vi "Begin.vi"(8 "error in":errorcluster) -> (0 "error out":errorcluster)   [LabVIEW 2015]
doc: "Called before other user functions, this VI is expected to open initial I/O refnums, load in file data, and do all program initialization. Notice that the <B>error out</B> terminal is simply used for data flow. Wiring it to other structures or subVIs ensures that this VI runs first."
uses:
  <vilib>/Rock Robotics/WPI/DriverStation/WPI_DriverStationRobotMode2.ctl
  <vilib>/Rock Robotics/WPI/Joystick/WPI_JoystickDeviceEnum.ctl
  <vilib>/Rock Robotics/SystemInterfaces/DIO/FPGA_DIOChannel.ctl
  <vilib>/Rock Robotics/SystemInterfaces/DIO/FPGA_DIORelayChannel.ctl
  <vilib>/Rock Robotics/WPI/Solenoid/WPI_SolenoidChannel.ctl
  <vilib>/Rock Robotics/SystemInterfaces/DIO/FPGA_DIOPWMChannel.ctl
  <vilib>/Rock Robotics/SystemInterfaces/spilib/spi_bus.ctl
  Robot Global Data.vi
  <vilib>/Rock Robotics/Network Tables/NT Write String Array.vi
  <vilib>/Rock Robotics/WPI/Switch/WPI_SwitchOpenLimit.vi
  <vilib>/Rock Robotics/WPI/Solenoid/WPI_SolenoidOpenDouble.vi
  <vilib>/Rock Robotics/WPI/Counter/WPI_CounterDigitalInputToDigitalSource.vi
  <vilib>/Rock Robotics/WPI/MotorControl/WPI_MotorControlOpenCANTalonSRX.vi
  <vilib>/Rock Robotics/WPI/MotorControl/WPI_MotorControlOpen VictorSP.vi
  <vilib>/Rock Robotics/WPI/Gyro/WPI_GyroXRS450_SPI_Open.vi
  <vilib>/Rock Robotics/WPI/Utilities/WPI_GetSetVariantRefNum.vi
  <vilib>/Rock Robotics/WPI/Accelerometer/InternalAccelerometer/WPI_AccelerometerInternalOpen.vi
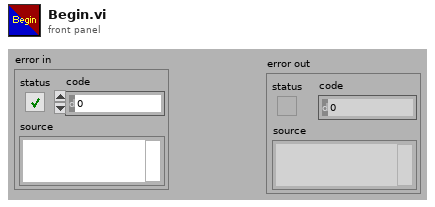
[diagram p1: front panel]
types:
  T1 = typedef "spi_bus.ctl" = enum16{"SPI On-Board, CS0", "SPI On-Board, CS1", "SPI On-Board, CS2", "SPI On-Board, CS3", "SPI MXP", "Invalid"}
  T2 = typedef "WPI_SolenoidChannel.ctl" = enum8{"Solenoid 0", "Solenoid 1", "Solenoid 2", "Solenoid 3", "Solenoid 4", "Solenoid 5", "Solenoid 6", "Solenoid 7", "Invalid"}
  T3 = typedef "FPGA_DIOPWMChannel.ctl" = enum8{"PWM 0", "PWM 1", "PWM 2", "PWM 3", "PWM 4", "PWM 5", "PWM 6", "PWM 7", "PWM 8", "PWM 9", "PWM MXP 0", "PWM MXP 1", "PWM MXP 2", "PWM MXP 3", "PWM MXP 4", "PWM MXP 5", "PWM MXP 6", "PWM MXP 7", "PWM MXP 8", "PWM MXP 9", "Invalid"}
  T4 = typedef "FPGA_DIOChannel.ctl" = enum8{"DIO 0", "DIO 1", "DIO 2", "DIO 3", "DIO 4", "DIO 5", "DIO 6", "DIO 7", "DIO 8", "DIO 9", "DIO MXP 0", "DIO MXP 1", "DIO MXP 2", "DIO MXP 3", "DIO MXP 4", "DIO MXP 5", "DIO MXP 6", "DIO MXP 7", "DIO MXP 8", "DIO MXP 9", "DIO MXP 10", "DIO MXP 11", "DIO MXP 12", "DIO MXP 13", "DIO MXP 14", "DIO MXP 15", "Invalid"}
  T5 = typedef "FPGA_DIORelayChannel.ctl" = enum8{"Relay 0", "Relay 1", "Relay 2", "Relay 3", "Invalid"}
  T6 = typedef "WPI_JoystickDeviceEnum.ctl" = enum16{"USB 0", "USB 1", "USB 2", "USB 3", "USB 4", "USB 5"}
  T7 = typedef "WPI_DriverStationRobotMode2.ctl" = enum16{"Autonomous Disabled", "Autonomous Enabled", "Teleop Disabled", "Teleop Enabled", "Disconnected", "Finish", "Test Disabled", "Test Enabled", "Emergency Stopped"}
  T8 = typedef "WPI_AccelerometerDevRef.ctl" = cluster{"DevStatus":errorcluster, "Scaling":T9, "Analog Channels":T10, "I2C Bus":T12, "SPI Bus":T1, "Accel Range":T13, "ADXL Axes":T14, "Handle":i32, "Device Address":u8, "Accel Type":enum16{"Analog", "ADXL345 I2C", "ADXL345 SPI", "Internal", "ADXL362 SPI"}}
  T9 = typedef "WPI_AccelerometerScaling.ctl" = cluster{"Gain (VoltsPerG)":dbl, "Center Voltage":dbl}
  T10 = typedef "WPI_AccelerometerAnalogChannels.ctl" = cluster{"X-Axis":T11, "Y-Axis":T11, "Z-Axis":T11}
  T11 = typedef "FPGA_AIChannel.ctl" = enum8{"AI 0", "AI 1", "AI 2", "AI 3", "AI MXP 0", "AI MXP 1", "AI MXP 2", "AI MXP 3", "Invalid"}
  T12 = typedef "i2c_bus.ctl" = enum16{"I2C On-Board", "I2C MXP", "Invalid"}
  T13 = typedef "ADXL345 Range.ctl" = u8
  T14 = typedef "WPI_AccelerometerADXL345 Axes.ctl" = cluster{"X-Axis":bool, "Y-Axis":bool, "Z-Axis":bool}
  T15 = typedef "WPI_CompressorDevRef.ctl" = cluster{"DevStatus":errorcluster, "Pneumatics Control Module":u8}
  T16 = typedef "WPI_MotorControlDeviceRef.ctl" = cluster{"DeviceStatus":errorcluster, "Type":T17, "PWM":cluster{"PWM Channel":T3, "DeadBand":T18}, "CAN":cluster{"Device Number":u8, "Control Mode":T19, "Semaphore":T20, "Max Vout":dbl, "TalonSRX Control Mode":T21}, "Invert":bool}
  T17 = typedef "WPI_MotorControlType.ctl" = enum16{"PWM", "CAN", "CANTalonSRX"}
  T18 = typedef "WPI_PWMDeadband.ctl" = cluster{"Name":string, "maxPositivePwm":i32, "minPositivePwm":i32, "centerPwm":i32, "maxNegativePwm":i32, "minNegativePwm":i32, "angularRange":u16}
  T19 = typedef "WPI_CANJaguar_ControlMode.ctl" = enum8{"Percent VBus", "Current", "Speed", "Position", "Voltage"}
  T20 = typedef "Semaphore RefNum" = refnum<k1>
  T21 = typedef "WPI_CANTalonSRX_APIControlMode.ctl" = enum8{"Percent VBus", "Speed", "Position", "Slave", "Unchanged / Invalid", "Voltage Compensation", "Current", "Motion Profile"}
  T22 = typedef "WPI_JoystickDevRef.ctl" = cluster{"Device":T6}
  T23 = typedef "WPI_DigitalInputDevRef.ctl" = cluster{"DevStatus":errorcluster, "DIO Channel":T4}
  T24 = typedef "WPI_SwitchDevRef.ctl" = cluster{"DevStatus":errorcluster, "DIO Channel":T4, "CntIndex":T25, "Normally Closed":bool}
  T25 = typedef "FPGA_CounterCtrSystemIndex.ctl" = enum8{"Ctr 0", "Ctr 1", "Ctr 2", "Ctr 3", "Ctr 4", "Ctr 5", "Ctr 6", "Ctr 7", "Invalid"}
  T26 = typedef "WPI_ServoDeviceRef.ctl" = cluster{"DeviceStatus":errorcluster, "PWM Channel":T3, "DeadBand":T18}
  T27 = typedef "WPI_RelayDevRef.ctl" = cluster{"DevStatus":errorcluster, "Relay Channel":T5, "Relay Direction":T28}
  T28 = typedef "WPI_RelayDirection.ctl" = enum16{"Both directions", "Forward only", "Reverse only"}
  T29 = typedef "WPI_SolenoidDevRef.ctl" = cluster{"DevStatus":errorcluster, "Pneumatics Control Module":u8, "Forward Solenoid Channel":T2, "Reverse Solenoid Channel":T2}
  T30 = typedef "FPGA_CounterEncoderSourceConvertionLVSourceType.ctl" = cluster{"DevStatus":errorcluster, "AnalogTriggerMode?":bool, "DigitalMode":cluster{"DIO Channel":T31}, "AnalogTriggerMode":cluster{"AnalogTriggerIndex":T32, "OutputType":T33}}
  T31 = typedef "FPGA_DIODigitalSourceChannel.ctl" = enum8{"DIO 0", "DIO 1", "DIO 2", "DIO 3", "DIO 4", "DIO 5", "DIO 6", "DIO 7", "DIO 8", "DIO 9", "DIO MXP 0", "DIO MXP 1", "DIO MXP 2", "DIO MXP 3", "DIO MXP 4", "DIO MXP 5", "DIO MXP 6", "DIO MXP 7", "DIO MXP 8", "DIO MXP 9", "DIO MXP 10", "DIO MXP 11", "DIO MXP 12", "DIO MXP 13", "DIO MXP 14", "DIO MXP 15", "Disabled"}
  T32 = typedef "FPGA_AnalogTriggerIndex.ctl" = enum8{"Trig 0", "Trig 1", "Trig 2", "Trig 3", "Trig 4", "Trig 5", "Trig 6", "Trig 7", "Invalid"}
  T33 = typedef "FPGA_AnalogTriggerOutType.ctl" = enum16{"InWindow", "TriggerState", "Rising", "Falling"}
  T34 = typedef "WPI_GyroDevRef.ctl" = cluster{"DevStatus":errorcluster, "Analog Channel":T11, "Offset":dbl, "Gain (VoltsPerDegree/Second)":dbl, "Gyro Type":enum16{"Analog", "XRS450"}, "Handle":i32, "SPI Bus":T1, "Device Found":bool, "Sample Rate":dbl, "Calibrate On Open":bool}
  T35 = typedef "WPI_EncoderDevRef.ctl" = cluster{"DevStatus":errorcluster, "EncoderIndex":T36, "CounterIndex":T25, "DistancePerCount":dbl, "Decoding Type":T37}
  T36 = typedef "FPGA_EncoderIdx.ctl" = enum8{"Enc 0", "Enc 1", "Enc 2", "Enc 3", "Enc 4", "Enc 5", "Enc 6", "Enc 7", "Invalid"}
  T37 = typedef "WPI_EncoderType.ctl" = enum16{"1x", "2x", "4x"}
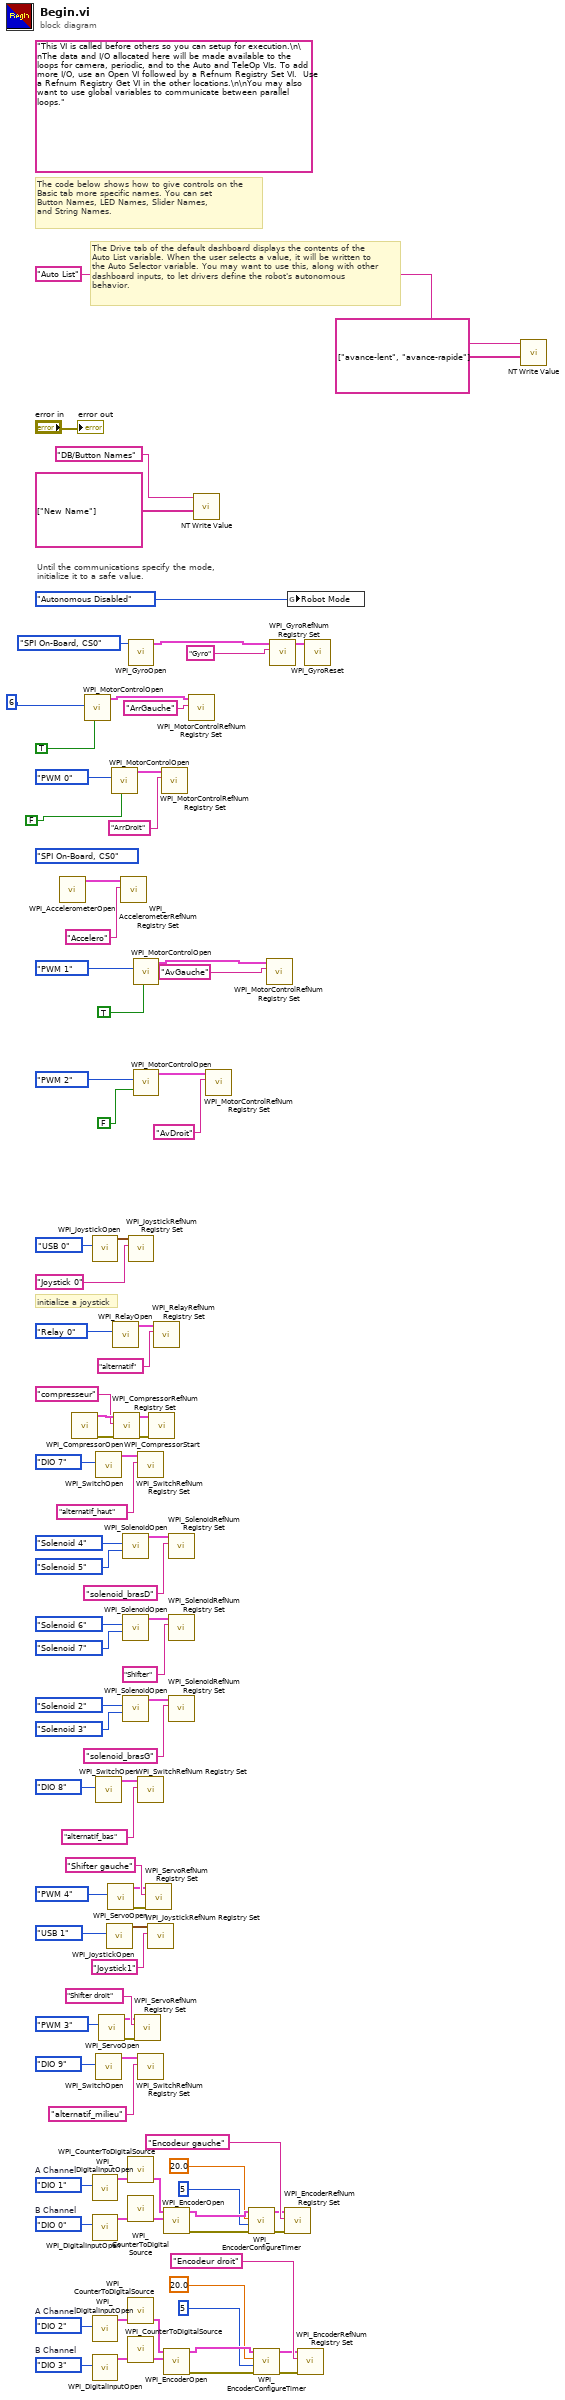
[diagram p0: block diagram]
diagram:
  (unwired) spi_bus."SPI On-Board, CS0" ("SPI Bus")
  w47 = FPGA_DIOChannel."DIO 0"  # B Channel
  w46 = FPGA_DIOChannel."DIO 1"  # A Channel
  w53 = FPGA_DIOChannel."DIO 3"  # B Channel
  w52 = FPGA_DIOChannel."DIO 2"  # A Channel
  (unwired) "This VI is called before others so you can setup for execution.\n\nThe data and I/O allocated here will be made available to the loops for camera, periodic, and to the Auto and TeleOp VIs. To add more I/O, use an Open VI followed by a Refnum Registry Set VI.  Use a Refnum Registry Get VI in the other locations.\n\nYou may also want to use global variables to communicate between parallel loops."
  # "The Drive tab of the default dashboard displays the contents of the\nAuto List variable. When the user selects a value, it will be written to\nthe Auto Selector variable. You may want to use this, along with other\ndashboard inputs, to let drivers define the robot's autonomous\nbehavior."
  # "The code below shows how to give controls on the\nBasic tab more specific names. You can set\nButton Names, LED Names, Slider Names,\nand String Names."
  # "initialize a joystick"
  # "Until the communications specify the mode,\ninitialize it to a safe value."
  n1 = call-poly <vilib>:"WPI_AccelerometerOpen.vi"() -> ("AccelerometerDevRef"=w36:T8)  [unwired: 10 in, 1 out]
  n2 = call <vilib>:"WPI_CompressorOpen.vi"() -> ("CompressorDevRef"=w65:T15, "error out"=w66:errorcluster)  [unwired: 14 in]
  n3 = call-poly <vilib>:"WPI_MotorControlOpen.vi"("Invert"=TRUE, "Device Number"=u8 6) -> ("MotorControlDeviceRef"=w22:T16)  [unwired: 8 in, 1 out]
  n4 = call <vilib>:"WPI_JoystickOpen.vi"("JoystickDevice"=WPI_JoystickDeviceEnum."USB 0") -> ("JoystickDevRef"=w95:T22)  [unwired: 10 in]
  n5 = call <vilib>:"WPI_DigitalInputOpen.vi"("DIO Channel"=w46) -> ("DigitalInputDevRef"=w43:T23)  [unwired: 1 in, 9 out]
  n6 = call <vilib>:"WPI_DigitalInputOpen.vi"("DIO Channel"=w47) -> ("DigitalInputDevRef"=w44:T23)  [unwired: 1 in, 9 out]
  n7 = call <vilib>:"WPI_DigitalInputOpen.vi"("DIO Channel"=w52) -> ("DigitalInputDevRef"=w49:T23)  [unwired: 1 in, 9 out]
  n8 = call <vilib>:"WPI_DigitalInputOpen.vi"("DIO Channel"=w53) -> ("DigitalInputDevRef"=w50:T23)  [unwired: 1 in, 9 out]
  n9 = call-poly <vilib>:"WPI_SwitchOpen.vi"("DIO Channel"=FPGA_DIOChannel."DIO 7") -> ("SwitchDevRef"=w85:T24)  [unwired: 9 in, 1 out]
  n10 = call-poly <vilib>:"WPI_SwitchOpen.vi"("DIO Channel"=FPGA_DIOChannel."DIO 8") -> ("SwitchDevRef"=w82:T24)  [unwired: 9 in, 1 out]
  n11 = call-poly <vilib>:"WPI_SwitchOpen.vi"("DIO Channel"=FPGA_DIOChannel."DIO 9") -> ("SwitchDevRef"=w75:T24)  [unwired: 9 in, 1 out]
  n12 = call <vilib>:"WPI_ServoOpen.vi"("PWM Channel"=FPGA_DIOPWMChannel."PWM 3" ("Front Left Motor")) -> ("error out"=w56:errorcluster, "ServoDeviceRef"=w59:T26)  [unwired: 9 in]
  n13 = call <vilib>:"WPI_JoystickOpen.vi"("JoystickDevice"=WPI_JoystickDeviceEnum."USB 1") -> ("JoystickDevRef"=w79:T22)  [unwired: 10 in]
  n14 = call <vilib>:"WPI_ServoOpen.vi"("PWM Channel"=FPGA_DIOPWMChannel."PWM 4" ("Front Left Motor")) -> ("error out"=w57:errorcluster, "ServoDeviceRef"=w58:T26)  [unwired: 9 in]
  n15 = call-poly <vilib>:"WPI_MotorControlOpen.vi"("Invert"=FALSE, "PWM Channel"=FPGA_DIOPWMChannel."PWM 0") -> ("MotorControlDeviceRef"=w19:T16)  [unwired: 8 in, 1 out]
  n16 = call <vilib>:"WPI_RelayOpen.vi"("Relay Channel"=FPGA_DIORelayChannel."Relay 0") -> ("RelayDevRef"=w74:T27)  [unwired: 9 in, 1 out]
  n17 = call <vilib>:"WPI_CompressorRefNum Registry Set.vi"("error in (no error)"=w66, "refnum name"="compresseur", "CompressorDevRef"=w65) -> ("error out"=w62:errorcluster, "CompressorDevRef"=w64:T15)  [unwired: 7 in]
  n18 = call <vilib>:"WPI_AccelerometerRefNum Registry Set.vi"("refnum name"="Accelero", "AccelerometerDevRef"=w36) -> ()  [unwired: 8 in, 2 out]
  n19 = call-poly <vilib>:"WPI_SolenoidOpen.vi"("Reverse Solenoid Channel"=WPI_SolenoidChannel."Solenoid 5", "Forward Solenoid Channel"=WPI_SolenoidChannel."Solenoid 4") -> ("SolenoidDevRef"=w12:T29)  [unwired: 8 in, 1 out]
  n20 = call-poly <vilib>:"WPI_SolenoidOpen.vi"("Reverse Solenoid Channel"=WPI_SolenoidChannel."Solenoid 7", "Forward Solenoid Channel"=WPI_SolenoidChannel."Solenoid 6") -> ("SolenoidDevRef"=w69:T29)  [unwired: 8 in, 1 out]
  n21 = call-poly <vilib>:"WPI_SolenoidOpen.vi"("Reverse Solenoid Channel"=WPI_SolenoidChannel."Solenoid 3", "Forward Solenoid Channel"=WPI_SolenoidChannel."Solenoid 2") -> ("SolenoidDevRef"=w72:T29)  [unwired: 8 in, 1 out]
  n22 = call-poly <vilib>:"WPI_CounterToDigitalSource.vi"("DigitalInputDevRef"=w43) -> ("Digital Source"=w5:T30)  [unwired: 6 out]
  n23 = call-poly <vilib>:"WPI_CounterToDigitalSource.vi"("DigitalInputDevRef"=w44) -> ("Digital Source"=w45:T30)  [unwired: 6 out]
  n24 = call-poly <vilib>:"WPI_CounterToDigitalSource.vi"("DigitalInputDevRef"=w49) -> ("Digital Source"=w4:T30)  [unwired: 6 out]
  n25 = call-poly <vilib>:"WPI_CounterToDigitalSource.vi"("DigitalInputDevRef"=w50) -> ("Digital Source"=w51:T30)  [unwired: 6 out]
  n26 = call-poly <vilib>:"WPI_GyroOpen.vi"("SPI Bus"=spi_bus."SPI On-Board, CS0") -> ("GyroDevRef"=w41:T34)  [unwired: 9 in, 1 out]
  n27 = call <vilib>:"WPI_JoystickRefNum Registry Set.vi"("refnum name"="Joystick 0", "JoystickDevRef"=w95) -> ()  [unwired: 8 in, 2 out]
  n28 = call-poly <vilib>:"WPI_MotorControlOpen.vi"("Invert"=TRUE, "PWM Channel"=FPGA_DIOPWMChannel."PWM 1") -> ("MotorControlDeviceRef"=w21:T16)  [unwired: 8 in, 1 out]
  n29 = call-poly <vilib>:"WPI_MotorControlOpen.vi"("Invert"=FALSE, "PWM Channel"=FPGA_DIOPWMChannel."PWM 2") -> ("MotorControlDeviceRef"=w20:T16)  [unwired: 8 in, 1 out]
  n30 = call <vilib>:"WPI_ServoRefNum Registry Set.vi"("error in (no error)"=w56, "refnum name"="Shifter droit", "ServoDeviceRef"=w59) -> ()  [unwired: 7 in, 2 out]
  n31 = call <vilib>:"WPI_SwitchRefNum Registry Set.vi"("refnum name"="alternatif_haut", "SwitchDevRef"=w85) -> ()  [unwired: 8 in, 2 out]
  n32 = call <vilib>:"WPI_SwitchRefNum Registry Set.vi"("refnum name"="alternatif_bas", "SwitchDevRef"=w82) -> ()  [unwired: 8 in, 2 out]
  n33 = call <vilib>:"WPI_SwitchRefNum Registry Set.vi"("refnum name"="alternatif_milieu", "SwitchDevRef"=w75) -> ()  [unwired: 8 in, 2 out]
  n34 = call <vilib>:"WPI_ServoRefNum Registry Set.vi"("error in (no error)"=w57, "refnum name"="Shifter gauche", "ServoDeviceRef"=w58) -> ()  [unwired: 7 in, 2 out]
  n35 = call <vilib>:"WPI_JoystickRefNum Registry Set.vi"("refnum name"="Joystick1", "JoystickDevRef"=w79) -> ()  [unwired: 8 in, 2 out]
  n36 = call <vilib>:"WPI_CompressorStart.vi"("error in (no error)"=w62, "CompressorDevRef"=w64) -> ()  [unwired: 8 in, 2 out]
  n37 = call <vilib>:"WPI_RelayRefNum Registry Set.vi"("refnum name"="alternatif", "RelayDevRef"=w74) -> ()  [unwired: 8 in, 2 out]
  n38 = call <vilib>:"WPI_MotorControlRefNum Registry Set.vi"("refnum name"="ArrDroit", "MotorControlDevRef"=w19) -> ()  [unwired: 8 in, 2 out]
  n39 = call <vilib>:"WPI_EncoderOpen.vi"("BSource"=w45, "ASource"=w5) -> ("error out"=w29:errorcluster, "EncoderDevRef"=w34:T35)  [unwired: 6 in, 2 out]
  n40 = call <vilib>:"WPI_EncoderOpen.vi"("BSource"=w51, "ASource"=w4) -> ("error out"=w26:errorcluster, "EncoderDevRef"=w28:T35)  [unwired: 6 in, 2 out]
  n41 = call <vilib>:"WPI_SolenoidRefNum Registry Set.vi"("refnum name"="solenoid_brasD", "SolenoidDevRef"=w12) -> ()  [unwired: 8 in, 2 out]
  n42 = call <vilib>:"WPI_SolenoidRefNum Registry Set.vi"("refnum name"="Shifter", "SolenoidDevRef"=w69) -> ()  [unwired: 8 in, 2 out]
  n43 = call <vilib>:"WPI_SolenoidRefNum Registry Set.vi"("refnum name"="solenoid_brasG", "SolenoidDevRef"=w72) -> ()  [unwired: 8 in, 2 out]
  n44 = call <vilib>:"WPI_MotorControlRefNum Registry Set.vi"("refnum name"="ArrGauche", "MotorControlDevRef"=w22) -> ()  [unwired: 8 in, 2 out]
  n45 = call-poly <vilib>:"NT Write Value.vi"("String Array"=string[] ["New Name"], "Name"="DB/Button Names") -> ()  [unwired: 9 in, 1 out]
  n46 = call <vilib>:"WPI_MotorControlRefNum Registry Set.vi"("refnum name"="AvDroit", "MotorControlDevRef"=w20) -> ()  [unwired: 8 in, 2 out]
  n47 = call <vilib>:"WPI_EncoderConfigureTimer.vi"("error in (no error)"=w29, "Number Samples to Average"=u8 5, "Minimum Rate"=20.0, "EncoderDevRef"=w34) -> ("error out"=w30:errorcluster, "EncoderDevRef"=w33:T35)  [unwired: 6 in]
  n48 = call <vilib>:"WPI_EncoderConfigureTimer.vi"("error in (no error)"=w26, "Number Samples to Average"=u8 5, "Minimum Rate"=20.0, "EncoderDevRef"=w28) -> ("error out"=w25:errorcluster, "EncoderDevRef"=w27:T35)  [unwired: 6 in]
  n49 = call <vilib>:"WPI_MotorControlRefNum Registry Set.vi"("refnum name"="AvGauche", "MotorControlDevRef"=w21) -> ()  [unwired: 8 in, 2 out]
  n50 = call <vilib>:"WPI_GyroRefNum Registry Set.vi"("refnum name"="Gyro", "GyroDevRef"=w41) -> ("GyroDevRef"=w37:T34)  [unwired: 8 in, 1 out]
  n51 = call <vilib>:"WPI_EncoderRefNum Registry Set.vi"("error in (no error)"=w30, "refnum name"="Encodeur gauche", "EncoderDevRef"=w33) -> ()  [unwired: 7 in, 2 out]
  n52 = global write "Robot Global Data.vi" "Robot Mode"(WPI_DriverStationRobotMode2."Autonomous Disabled" ("Robot Mode")) -> ()
  n53 = call <vilib>:"WPI_EncoderRefNum Registry Set.vi"("error in (no error)"=w25, "refnum name"="Encodeur droit", "EncoderDevRef"=w27) -> ()  [unwired: 7 in, 2 out]
  n54 = call <vilib>:"WPI_GyroReset.vi"("GyroDevRef"=w37) -> ()  [unwired: 9 in, 2 out]
  n55 = call-poly <vilib>:"NT Write Value.vi"("String Array"=string[] ["avance-lent", "avance-rapide"], "Name"="Auto List") -> ()  [unwired: 9 in, 1 out]
  "error out" <- "error in"
